vi "Get Child Items.vi"(8 "error in (no error)":errorcluster, 11 "item ref in":T1 format="%.0x") -> (0 "error out":errorcluster, 2 "child item refs out":u64[](array[numeric]), 3 "item ref out":T1 format="%.0x")   [LabVIEW 2018, in "FPGA Addon System Explorer.lvlib"]
uses:
  FPGA Addon System Explorer.lvlib
  <vilib>/NI Veristand/Custom Device API/Custom Device Item Ref.ctl
  NationalInstruments.VeriStand.SystemDefinitionAPI
  <vilib>/NI Veristand/Custom Device API/Custom Device API.lvlib
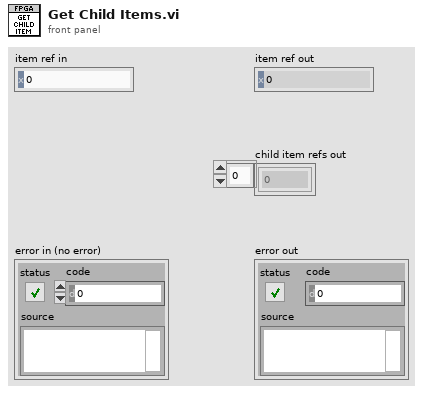
[diagram p1: front panel]
types:
  T1 = typedef "Custom Device API.lvlib/Custom Device Item Ref.ctl" = u64
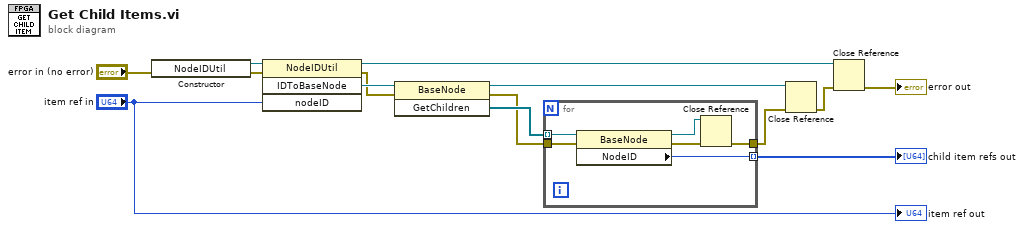
[diagram p0: block diagram]
diagram:
  n1 = constructor class="NodeIDUtil"(error in="error in (no error)") -> (reference out=w12:refnum<k24>, error out=w11:errorcluster)  [unwired: 2 in, 1 out]
  n2 = invoke class="NodeIDUtil" method="IDToBaseNode"(reference=w12, error in=w11, "nodeID"="item ref in") -> (reference out=w2:refnum<k24>, error out=w9:errorcluster, "IDToBaseNode"=w14:refnum<k24>)  [unwired: 1 in, 1 out]
  n3 = invoke class="BaseNode" method="GetChildren"(reference=w14, error in=w9) -> (reference out=w4:refnum<k24>, error out=w7:errorcluster, "GetChildren"=w8:refnum<k24>[])  [unwired: 1 in]
  n4 = for {
    tunnel: w8 -> [w20] mode=indexing
    tunnel: w7 -> [w19]
    tunnel: [w18] -> w6 mode=indexing
    tunnel: [w15] -> w5
    n5 = property class="BaseNode"(reference=w20, error in=w19) -> (reference out=w16:refnum<k24>, error out=w17:errorcluster, "NodeID"=w18:u64)
    n6 = Close Reference(reference=w16, error in (no error)=w17) -> (error out=w15:errorcluster)
  }
  "child item refs out" <- w6
  n7 = Close Reference(reference=w4, error in (no error)=w5) -> (error out=w3:errorcluster)
  n8 = Close Reference(reference=w2, error in (no error)=w3) -> (error out=→"error out":errorcluster)
  "item ref out" <- "item ref in"
